vi "Database Module.vi"(8 "error in":errorcluster) -> (0 "error out":errorcluster)   [LabVIEW 2018, in "Database.lvlib"]
doc: "This is the top level of the database module (a free running module of the Car Wash simulator). \n\nIt is closed using a user event. It communicates with the other modules using a queue based API which has comms modules that can be swapped if required."
uses:
  Database.lvlib
  Classes/database.lvclass
  Private Controls/Module Data Cluster.ctl
  Private Controls/Module Action.ctl
  <vilib>/addons/database/_DB Variant To Data/Database Variant To Data.xnode
  Base Controller/Controller.lvlib
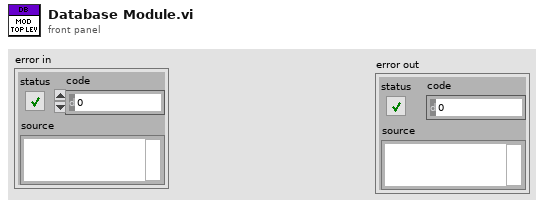
[diagram p1: front panel]
types:
  T1 = cluster{"Step Duration":string, "Station":string, "Wash Step":string}
  T2 = typedef "Database.lvlib/Module Data Cluster.ctl" = cluster{"Variant":variant, "action":T3}
  T3 = typedef "Database.lvlib/Module Action.ctl" = enum16{"error", "exit", "init", "Read Database Record", "Update record", "Insert Record", "Release Connection", "Login"}
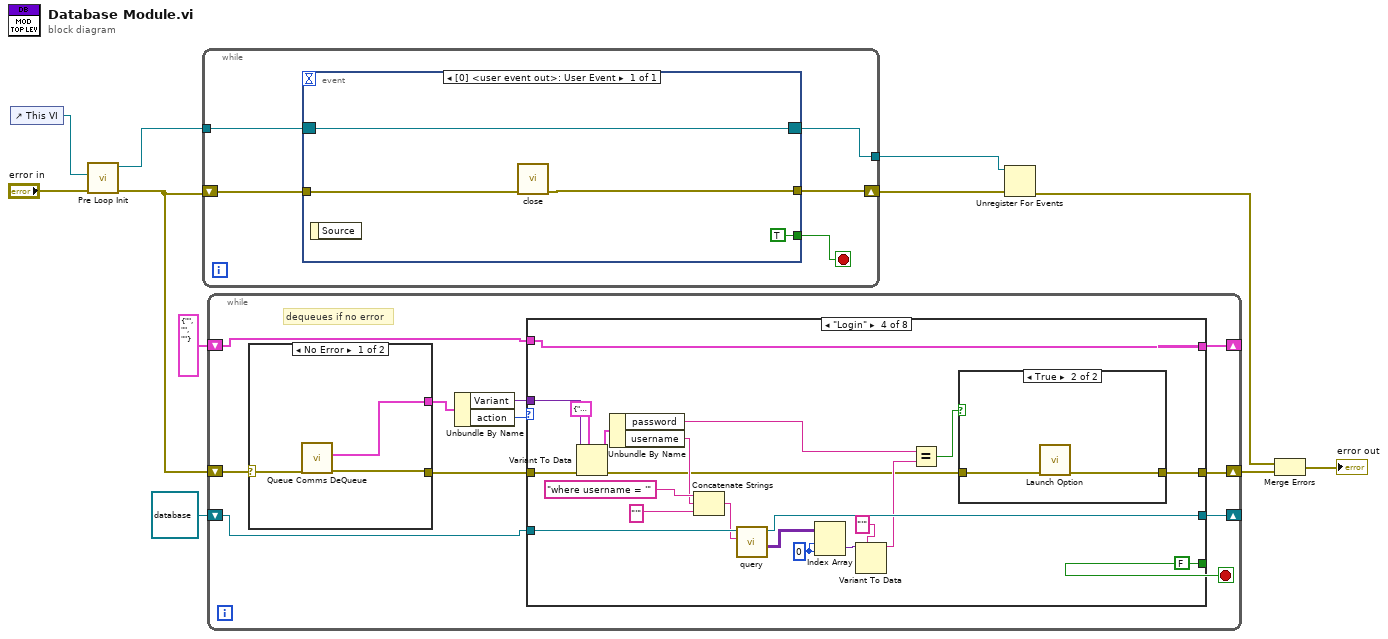
[diagram p0: block diagram]
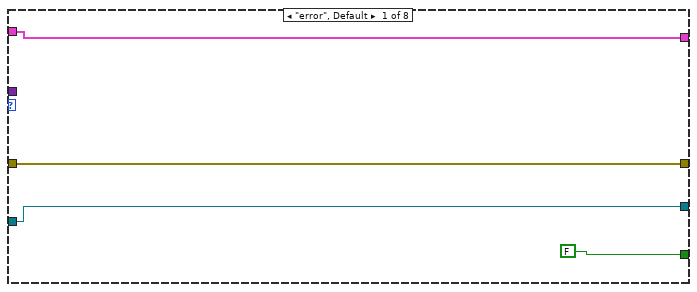
[diagram p2: hidden frame]
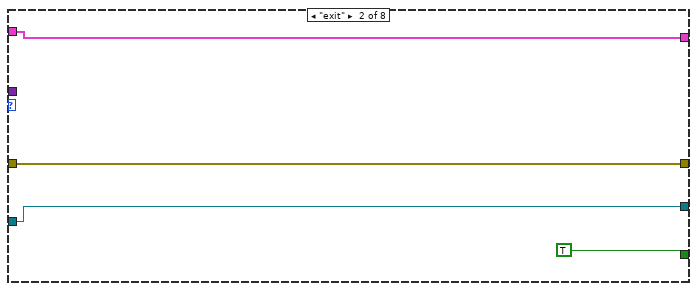
[diagram p3: hidden frame]
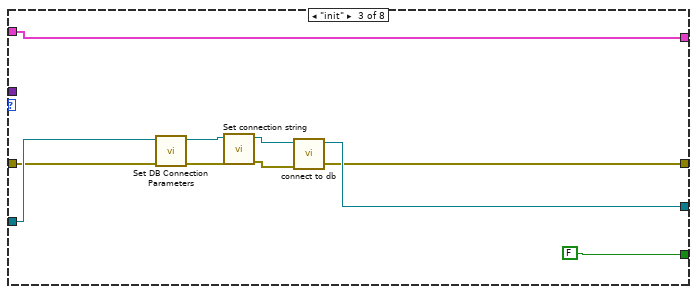
[diagram p4: hidden frame]
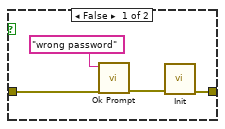
[diagram p5: hidden frame]
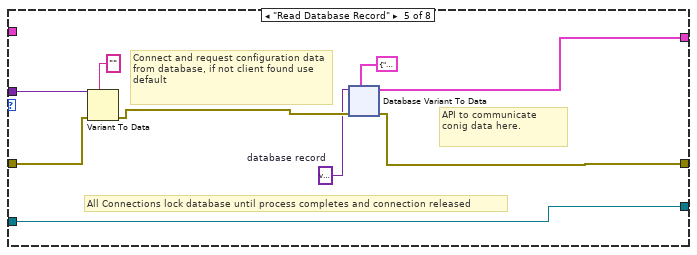
[diagram p6: hidden frame]
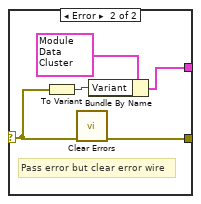
[diagram p10: hidden frame]
diagram:
  n1 = control-ref of="This VI"() -> (w11:refnum<vi>)
  n2 = call "Pre Loop Init.vi"("error in"="error in", "Ref In"=w11) -> ("error out"=w8:errorcluster, "Event Registration Refnum"=w10:refnum<event-registration>)  [unwired: 8 in]
  n3 = while {
    shift-right: [w15] -> w7
    shift-left: w8 -> [w16]
    tunnel: w10 -> [w14]
    tunnel: [w12] -> w6
    stop <- w13 stop-if-true
    n4 = event shown="[0] <user event out>: User Event" {
      selector: w14 -> [w17]
      dyn-events: [w17] -> w12
      timeout: _ -> [_]
      tunnel: w16 -> [w20]
      tunnel: [w19] -> w15
      tunnel: [TRUE] -> w13
      event User Event {
        n5 = event-data() -> ()  [unwired: 1 in, 1 out]
        n6 = call "close.vi"("error in"=w20) -> ("error out"=w19:errorcluster)  [unwired: 10 in]
      }
    }
  }
  n7 = while {
    shift-right: [w27] -> w5
    shift-left: w8 -> [w31]
    shift-right: [w24] -> _
    shift-left: T1 {"Step Duration"="", "Station"="", "Wash Step"=""} ("data") -> [w23]
    shift-right: [w22] -> _
    shift-left: refnum<class "database.lvclass"> refnum ("database out") -> [w21]
    stop <- w25 stop-if-true
    # "dequeues if no error"
    n8 = case shown="No Error" w31 {
      selector: w31 -> [w132 w137]
      tunnel: [w131 w133] -> w30
      tunnel: [w130 w136] -> w26
      frame No Error {
        n9 = call "Queue Comms DeQueue.vi"("error in"=w132) -> ("error out"=w130:errorcluster, "element"=w131:T2)  [unwired: 9 in]
      }
      frame Error {
        # "Pass error but clear error wire"
        n10 = To Variant(anything=w137) -> (Variant=w134:variant)
        n11 = call <vilib>:"Clear Errors.vi"("error in (no error)"=w137) -> ("error out"=w136:errorcluster)  [unwired: 5 in, 1 out]
        n12 = Bundle By Name(cluster=T2 {"Variant"=variant, "action"=enum."error"} ("element"), "Variant"=w134) -> (w133:T2)
      }
    }
    n13 = Unbundle By Name(w30) -> ("Variant"=w28:variant, "action"=w29:T3)
    n14 = case shown="\"Login\"" w29 {
      tunnel: w28 -> [_ _ _ w67 w85 _ _ _]
      tunnel: [w35 w39 w40 w50 w78 w123 w126 w129] -> w27
      tunnel: w26 -> [w35 w39 w41 w61 w81 w123 w126 w129]
      tunnel: [FALSE TRUE FALSE FALSE _ _ _ _] -> w25
      tunnel: [w33 w37 w48 w70 w82 w122 w125 w128] -> w24
      tunnel: w23 -> [w33 w37 w48 w70 _ w122 w125 w128]
      tunnel: [w32 w36 w43 w68 w77 w121 w124 w127] -> w22
      tunnel: w21 -> [w32 w36 w42 w69 w77 w121 w124 w127]
      frame "error", Default {
      }
      frame "exit" {
      }
      frame "init" {
        n15 = call-dynamic "Set DB Connection Parameters.vi"("error in (no error)"=w41, "database in"=w42) -> ("error out"=w45:errorcluster, "database out"=w47:refnum<class "database.lvclass">)  [unwired: 8 in]
        n16 = call-dynamic "Set connection string.vi"("error in (no error)"=w45, "database in"=w47) -> ("error out"=w44:errorcluster, "database out"=w46:refnum<class "database.lvclass">)  [unwired: 8 in]
        n17 = call-dynamic "connect to db.vi"("error in (no error)"=w44, "database in"=w46) -> ("error out"=w40:errorcluster, "database out"=w43:refnum<class "database.lvclass">)  [unwired: 8 in]
      }
      frame "Login" {
        w65 = 0 ("disabled index (col)")
        n18 = Variant To Data(error in=w61, type=cluster{"password":string, "username":string} {"password"="", "username"=""}, Variant=w67) -> (data=w62:cluster{"password":string, "username":string}, error out=w51:errorcluster)
        n19 = Unbundle By Name(w62) -> ("password"=w54:string, "username"=w58:string)
        n20 = Concatenate Strings("where username = '" ("condition"), w58, "'" ("condition")) -> (w56:string)
        n21 = call-dynamic "query.vi"("condition"=w56, "database in"=w69) -> ("data"=w64:variant[][], "database out"=w68:refnum<class "database.lvclass">)  [unwired: 7 in, 1 out]
        n22 = Index Array(array=w64, index (row)=w65, index (col)=w65) -> (element=w66:variant)
        n23 = Variant To Data(type="'" ("condition"), Variant=w66) -> (data=w53:string)  [unwired: 1 in, 1 out]
        n24 = Equal?(x=w54, y=w53) -> (x = y?=w52:bool)
        n25 = case shown="True" w52 {
          tunnel: w51 -> [w73 w76]
          tunnel: [w74 w75] -> w50
          frame False {
            n26 = call "Ok Prompt.vi"("error in"=w73, "Message"="wrong password") -> ("error out"=w72:errorcluster)  [unwired: 9 in]
            n27 = call "Init.vi"("error in"=w72) -> ("error out"=w74:errorcluster)  [unwired: 10 in]
          }
          frame True {
            n28 = call "Launch Option.vi"("error in"=w76) -> ("error out"=w75:errorcluster)  [unwired: 10 in]
          }
        }
      }
      frame "Read Database Record" {
        w79 = variant  # database record
        # "API to communicate conig data here."
        # "All Connections lock database until process completes and connection released"
        # "Connect and request configuration data from database, if not client found use default"
        n29 = Variant To Data(error in=w81, type="" ("client"), Variant=w85) -> (error out=w80:errorcluster)  [unwired: 1 out]
        n30 = xnode "Database Variant To Data"("database variant"=w79, "error in (no error)"=w80, "type"=T1 {"Step Duration"="", "Station"="", "Wash Step"=""} ("Database Record")) -> ("data"=w82:T1, "error out"=w78:errorcluster)
      }
      frame "Release Connection" {
        # "[Covers : SD7]"
        # "at the end of every connection to the database, release the connection"
      }
      frame "Update record" {
      }
      frame "Insert Record" {
      }
    }
  }
  n31 = Unregister For Events(event registration refnum=w6, error in=w7) -> (error out=w3:errorcluster)
  n32 = Merge Errors(w3, w5) -> (→"error out":errorcluster)
